vi "DIO_type-casting_test.vi"() -> ()   [LabVIEW 2016]
uses:
  Type_Defs/Digital_Out_1.ctl
  Type_Defs/Digital_Out_2.ctl
  Type_Defs/Digital_In_1.ctl
  Type_Defs/Digital_In_2.ctl
panel:
  out "test 2":T5
  out "TF 2":bool
  out "TF 1":bool
  out "test 1":T5
  out "Origonal":T5
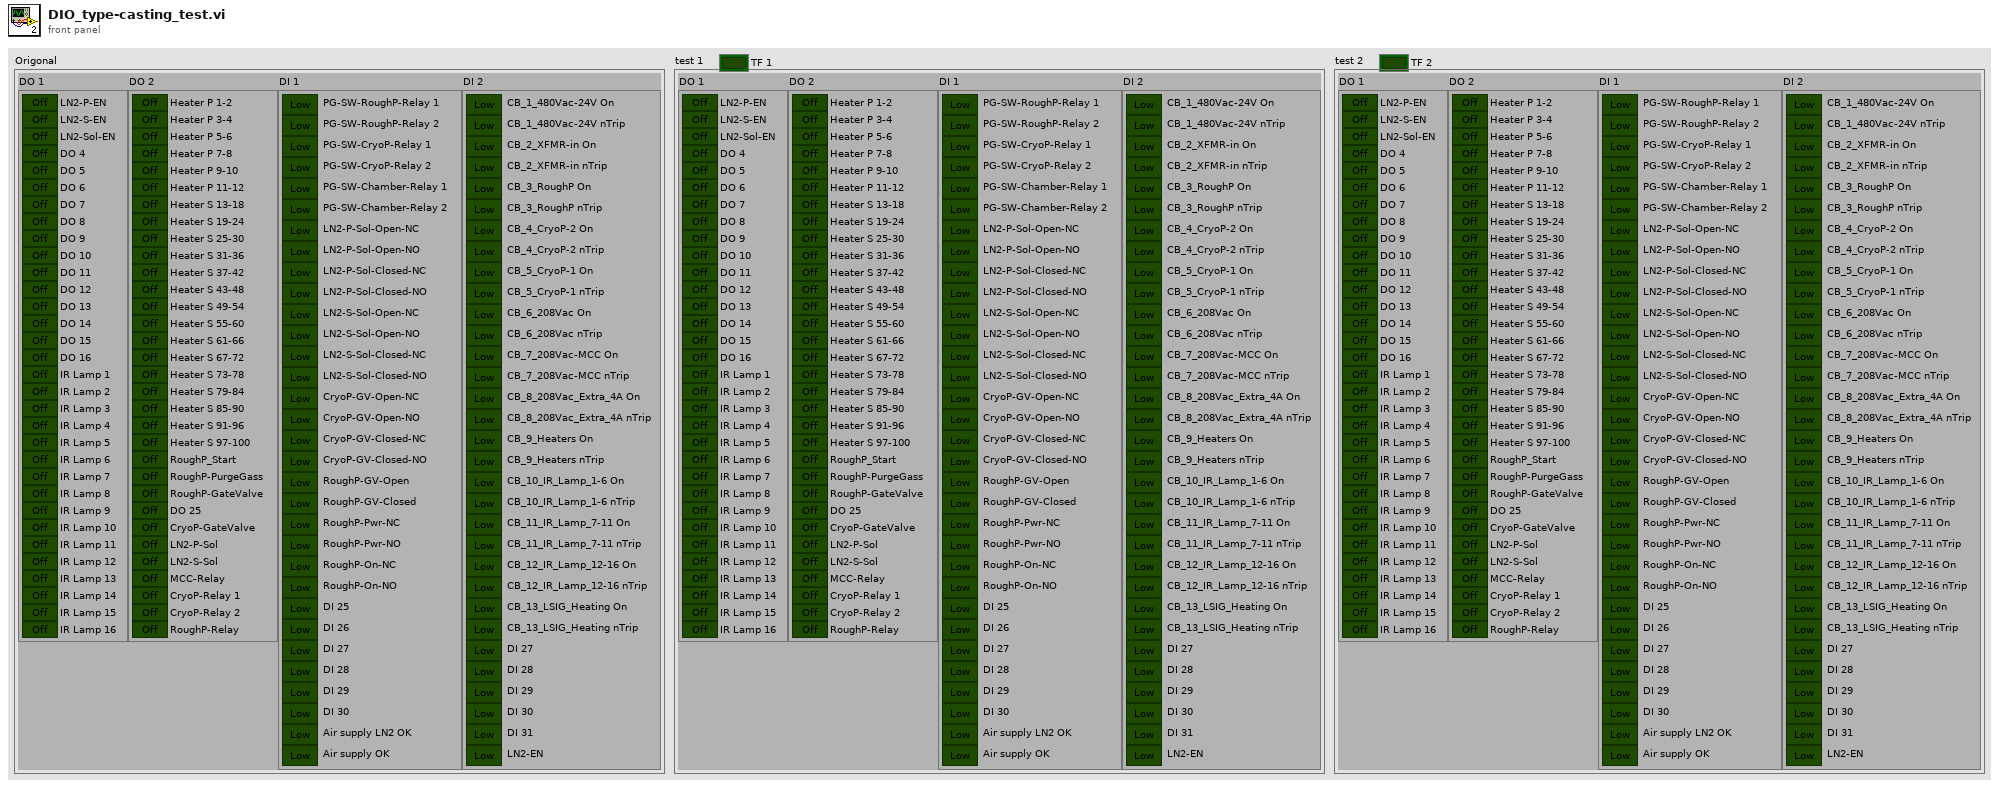
[diagram p1: front panel]
types:
  T1 = typedef "Digital_Out_1.ctl" = cluster{"LN2-P-EN":bool, "LN2-S-EN":bool, "LN2-Sol-EN":bool, "DO 4":bool, "DO 5":bool, "DO 6":bool, "DO 7":bool, "DO 8":bool, "DO 9":bool, "DO 10":bool, "DO 11":bool, "DO 12":bool, "DO 13":bool, "DO 14":bool, "DO 15":bool, "DO 16":bool, "IR Lamp 1":bool, "IR Lamp 2":bool, "IR Lamp 3":bool, "IR Lamp 4":bool, "IR Lamp 5":bool, "IR Lamp 6":bool, "IR Lamp 7":bool, "IR Lamp 8":bool, "IR Lamp 9":bool, "IR Lamp 10":bool, "IR Lamp 11":bool, "IR Lamp 12":bool, "IR Lamp 13":bool, "IR Lamp 14":bool, "IR Lamp 15":bool, "IR Lamp 16":bool}
  T2 = typedef "Digital_Out_2.ctl" = cluster{"Heater P 1-2":bool, "Heater P 3-4":bool, "Heater P 5-6":bool, "Heater P 7-8":bool, "Heater P 9-10":bool, "Heater P 11-12":bool, "Heater S 13-18":bool, "Heater S 19-24":bool, "Heater S 25-30":bool, "Heater S 31-36":bool, "Heater S 37-42":bool, "Heater S 43-48":bool, "Heater S 49-54":bool, "Heater S 55-60":bool, "Heater S 61-66":bool, "Heater S 67-72":bool, "Heater S 73-78":bool, "Heater S 79-84":bool, "Heater S 85-90":bool, "Heater S 91-96":bool, "Heater S 97-100":bool, "RoughP_Start":bool, "RoughP-PurgeGass":bool, "RoughP-GateValve":bool, "DO 25":bool, "CryoP-GateValve":bool, "LN2-P-Sol":bool, "LN2-S-Sol":bool, "MCC-Relay":bool, "CryoP-Relay 1":bool, "CryoP-Relay 2":bool, "RoughP-Relay":bool}
  T3 = typedef "Digital_In_1.ctl" = cluster{"PG-SW-RoughP-Relay 1":bool, "PG-SW-RoughP-Relay 2":bool, "PG-SW-CryoP-Relay 1":bool, "PG-SW-CryoP-Relay 2":bool, "PG-SW-Chamber-Relay 1":bool, "PG-SW-Chamber-Relay 2":bool, "LN2-P-Sol-Open-NC":bool, "LN2-P-Sol-Open-NO":bool, "LN2-P-Sol-Closed-NC":bool, "LN2-P-Sol-Closed-NO":bool, "LN2-S-Sol-Open-NC":bool, "LN2-S-Sol-Open-NO":bool, "LN2-S-Sol-Closed-NC":bool, "LN2-S-Sol-Closed-NO":bool, "CryoP-GV-Open-NC":bool, "CryoP-GV-Open-NO":bool, "CryoP-GV-Closed-NC":bool, "CryoP-GV-Closed-NO":bool, "RoughP-GV-Open":bool, "RoughP-GV-Closed":bool, "RoughP-Pwr-NC":bool, "RoughP-Pwr-NO":bool, "RoughP-On-NC":bool, "RoughP-On-NO":bool, "DI 25":bool, "DI 26":bool, "DI 27":bool, "DI 28":bool, "DI 29":bool, "DI 30":bool, "Air supply LN2 OK":bool, "Air supply OK":bool}
  T4 = typedef "Digital_In_2.ctl" = cluster{"CB_1_480Vac-24V On":bool, "CB_1_480Vac-24V nTrip":bool, "CB_2_XFMR-in On":bool, "CB_2_XFMR-in nTrip":bool, "CB_3_RoughP On":bool, "CB_3_RoughP nTrip":bool, "CB_4_CryoP-2 On":bool, "CB_4_CryoP-2 nTrip":bool, "CB_5_CryoP-1 On":bool, "CB_5_CryoP-1 nTrip":bool, "CB_6_208Vac On":bool, "CB_6_208Vac nTrip":bool, "CB_7_208Vac-MCC On":bool, "CB_7_208Vac-MCC nTrip":bool, "CB_8_208Vac_Extra_4A On":bool, "CB_8_208Vac_Extra_4A nTrip":bool, "CB_9_Heaters On":bool, "CB_9_Heaters nTrip":bool, "CB_10_IR_Lamp_1-6 On":bool, "CB_10_IR_Lamp_1-6 nTrip":bool, "CB_11_IR_Lamp_7-11 On":bool, "CB_11_IR_Lamp_7-11 nTrip":bool, "CB_12_IR_Lamp_12-16 On":bool, "CB_12_IR_Lamp_12-16 nTrip":bool, "CB_13_LSIG_Heating On":bool, "CB_13_LSIG_Heating nTrip":bool, "DI 27":bool, "DI 28":bool, "DI 29":bool, "DI 30":bool, "DI 31":bool, "LN2-EN":bool}
  T5 = cluster{"DO 1":T1, "DO 2":T2, "DI 1":T3, "DI 2":T4}
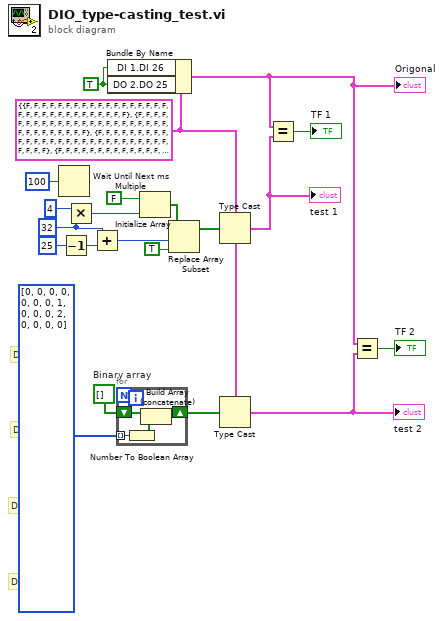
[diagram p0: block diagram]
diagram:
  w3 = bool[] []  # Binary array
  w15 = 32 ("dimension size")
  w1 = TRUE ("DO 2.DO 25")
  w6 = T5 {"DO 1"={"LN2-P-EN"=FALSE, "LN2-S-EN"=FALSE, "LN2-Sol-EN"=FALSE, "DO 4"=FALSE, "DO 5"=FALSE, "DO 6"=FALSE, "DO 7"=FALSE, "DO 8"=FALSE, "DO 9"=FALSE, "DO 10"=FALSE, "DO 11"=FALSE, "DO 12"=FALSE, "DO 13"=FALSE, "DO 14"=FALSE, "DO 15"=FALSE, "DO 16"=FALSE, "IR Lamp 1"=FALSE, "IR Lamp 2"=FALSE, "IR Lamp 3"=FALSE, "IR Lamp 4"=FALSE, "IR Lamp 5"=FALSE, "IR Lamp 6"=FALSE, "IR Lamp 7"=FALSE, "IR Lamp 8"=FALSE, "IR Lamp 9"=FALSE, "IR Lamp 10"=FALSE, "IR Lamp 11"=FALSE, "IR Lamp 12"=FALSE, "IR Lamp 13"=FALSE, "IR Lamp 14"=FALSE, "IR Lamp 15"=FALSE, "IR Lamp 16"=FALSE}, "DO 2"={"Heater P 1-2"=FALSE, "Heater P 3-4"=FALSE, "Heater P 5-6"=FALSE, "Heater P 7-8"=FALSE, "Heater P 9-10"=FALSE, "Heater P 11-12"=FALSE, "Heater S 13-18"=FALSE, "Heater S 19-24"=FALSE, "Heater S 25-30"=FALSE, "Heater S 31-36"=FALSE, "Heater S 37-42"=FALSE, "Heater S 43-48"=FALSE, "Heater S 49-54"=FALSE, "Heater S 55-60"=FALSE, "Heater S 61-66"=FALSE, "Heater S 67-72"=FALSE, "Heater S 73-78"=FALSE, "Heater S 79-84"=FALSE, "Heater S 85-90"=FALSE, "Heater S 91-96"=FALSE, "Heater S 97-100"=FALSE, "RoughP_Start"=FALSE, "RoughP-PurgeGass"=FALSE, "RoughP-GateValve"=FALSE, "DO 25"=FALSE, "CryoP-GateValve"=FALSE, "LN2-P-Sol"=FALSE, "LN2-S-Sol"=FALSE, "MCC-Relay"=FALSE, "CryoP-Relay 1"=FALSE, "CryoP-Relay 2"=FALSE, "RoughP-Relay"=FALSE}, "DI 1"={"PG-SW-RoughP-Relay 1"=FALSE, "PG-SW-RoughP-Relay 2"=FALSE, "PG-SW-CryoP-Relay 1"=FALSE, "PG-SW-CryoP-Relay 2"=FALSE, "PG-SW-Chamber-Relay 1"=FALSE, "PG-SW-Chamber-Relay 2"=FALSE, "LN2-P-Sol-Open-NC"=FALSE, "LN2-P-Sol-Open-NO"=FALSE, "LN2-P-Sol-Closed-NC"=FALSE, "LN2-P-Sol-Closed-NO"=FALSE, "LN2-S-Sol-Open-NC"=FALSE, "LN2-S-Sol-Open-NO"=FALSE, "LN2-S-Sol-Closed-NC"=FALSE, "LN2-S-Sol-Closed-NO"=FALSE, "CryoP-GV-Open-NC"=FALSE, "CryoP-GV-Open-NO"=FALSE, "CryoP-GV-Closed-NC"=FALSE, "CryoP-GV-Closed-NO"=FALSE, "RoughP-GV-Open"=FALSE, "RoughP-GV-Closed"=FALSE, "RoughP-Pwr-NC"=FALSE, "RoughP-Pwr-NO"=FALSE, "RoughP-On-NC"=FALSE, "RoughP-On-NO"=FALSE, "DI 25"=FALSE, "DI 26"=FALSE, "DI 27"=FALSE, "DI 28"=FALSE, "DI 29"=FALSE, "DI 30"=FALSE, "Air supply LN2 OK"=FALSE, "Air supply OK"=FALSE}, "DI 2"={"CB_1_480Vac-24V On"=FALSE, "CB_1_480Vac-24V nTrip"=FALSE, "CB_2_XFMR-in On"=FALSE, "CB_2_XFMR-in nTrip"=FALSE, "CB_3_RoughP On"=FALSE, "CB_3_RoughP nTrip"=FALSE, "CB_4_CryoP-2 On"=FALSE, "CB_4_CryoP-2 nTrip"=FALSE, "CB_5_CryoP-1 On"=FALSE, "CB_5_CryoP-1 nTrip"=FALSE, "CB_6_208Vac On"=FALSE, "CB_6_208Vac nTrip"=FALSE, "CB_7_208Vac-MCC On"=FALSE, "CB_7_208Vac-MCC nTrip"=FALSE, "CB_8_208Vac_Extra_4A On"=FALSE, "CB_8_208Vac_Extra_4A nTrip"=FALSE, "CB_9_Heaters On"=FALSE, "CB_9_Heaters nTrip"=FALSE, "CB_10_IR_Lamp_1-6 On"=FALSE, "CB_10_IR_Lamp_1-6 nTrip"=FALSE, "CB_11_IR_Lamp_7-11 On"=FALSE, "CB_11_IR_Lamp_7-11 nTrip"=FALSE, "CB_12_IR_Lamp_12-16 On"=FALSE, "CB_12_IR_Lamp_12-16 nTrip"=FALSE, "CB_13_LSIG_Heating On"=FALSE, "CB_13_LSIG_Heating nTrip"=FALSE, "DI 27"=FALSE, "DI 28"=FALSE, "DI 29"=FALSE, "DI 30"=FALSE, "DI 31"=FALSE, "LN2-EN"=FALSE}}
  # "Di2: 16"
  # "Di1: 12"
  # "Do2: 8"
  # "Do1: 4"
  n1 = Wait Until Next ms Multiple(millisecond multiple=u32 100) -> ()  [unwired: 1 out]
  n2 = Decrement(x=25 ("y")) -> (x-1=w13:i32)
  n3 = Multiply(x=4, y=w15) -> (x*y=w19:i32)
  n4 = Add(x=w15, y=w13) -> (x+y=w16:i32)
  n5 = Bundle By Name(cluster=w6, "DI 1.DI 26"=w1, "DO 2.DO 25"=w1) -> (w5:T5)
  "Origonal" <- w5
  n6 = for {
    tunnel: u8[] [0, 0, 0, 0, 0, 0, 0, 1, 0, 0, 0, 2, 0, 0, 0, 0] -> [w23] mode=indexing
    shift-right: [w24] -> w2
    shift-left: w3 -> [w25]
    n7 = Number To Boolean Array(number=w23) -> (Boolean array=w22:bool[])
    n8 = Build Array (concatenate)(w25, w22) -> (w24:bool[])
  }
  n9 = Initialize Array(FALSE, w19) -> (w17:bool[])
  n10 = Replace Array Subset(array=w17, new element=TRUE ("new element/subarray"), index=w16) -> (w11:bool[])
  n11 = Type Cast(type=w6, x=w11) -> (*(type *) &x=w10:T5)
  "test 1" <- w10
  n12 = Type Cast(type=w6, x=w2) -> (*(type *) &x=w7:T5)
  "test 2" <- w7
  n13 = Equal?(x=w5, y=w10) -> (x = y?=→"TF 1":bool)
  n14 = Equal?(x=w5, y=w7) -> (x = y?=→"TF 2":bool)
